vi "Build Channel Group Info.vi"(8 "Channel Data Reference":i32, 9 "Channel Groups in":T2(array[cluster]), 10 "Group Name":string, 11 "Channel Type":T1=enum."Input/Read") -> (0 "Group Index":i32, 1 "Channel Groups out":T2(array[cluster]))   [LabVIEW 2026, in "NIDMM Deployment Hooks.lvlib"]
uses:
  NIDMM Deployment Hooks.lvlib
  Types/Channel Mode.ctl
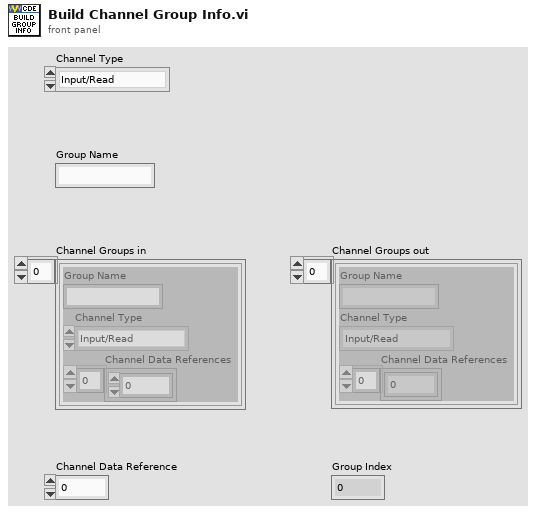
[diagram p1: front panel]
types:
  T1 = typedef "NIDMM Deployment Hooks.lvlib/Channel Mode.ctl" = enum16{"Output/Write", "Input/Read", "Input/ReadWrite"}
  T2 = cluster{"Group Name":string, "Channel Type":T1, "Channel Data References":i32[]}[]
  T3 = cluster{"Group Name":string, "Channel Type":T1, i32[]}
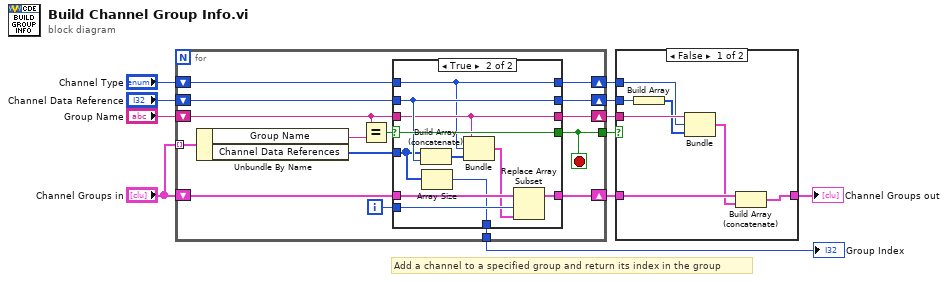
[diagram p0: block diagram]
diagram:
  # "Add a channel to a specified group and return its index in the group"
  n1 = for {
    tunnel: "Channel Groups in" -> [w26] mode=indexing
    shift-right: [w19] -> w8
    shift-left: "Channel Groups in" -> [w24]
    tunnel: [w17] -> w7
    shift-right: [w16] -> w11
    shift-left: "Channel Data Reference" -> [w22]
    shift-right: [w15] -> w10
    shift-left: "Group Name" -> [w20]
    shift-right: [w13] -> w2
    shift-left: "Channel Type" -> [w14]
    tunnel: [w12] -> w1
    i -> [w21]
    stop <- w17 stop-if-true
    n2 = Unbundle By Name(w26) -> ("Group Name"=w25:string, "Channel Data References"=w23:i32[])
    n3 = Equal?(x=w20, y=w25) -> (x = y?=w18:bool)
    n4 = case shown="True" w18 {
      selector: w18 -> [w30 w38]
      tunnel: w24 -> [w31 w42]
      tunnel: w23 -> [_ w33]
      tunnel: w22 -> [w29 w37]
      tunnel: w21 -> [_ w41]
      tunnel: w20 -> [w28 w36]
      tunnel: [w31 w39] -> w19
      tunnel: [w30 w38] -> w17
      tunnel: [w29 w37] -> w16
      tunnel: [w28 w36] -> w15
      tunnel: w14 -> [w27 w35]
      tunnel: [w27 w35] -> w13
      tunnel: [_ w32] -> w12
      frame False {
      }
      frame True {
        n5 = Build Array (concatenate)(w33, w37) -> (w34:i32[])
        n6 = Array Size(array=w33) -> (size(s)=w32:i32)
        n7 = Bundle("Group Name"=w36, "Channel Type"=w35, w34) -> (w40:T3)  [unwired: 1 in]
        n8 = Replace Array Subset(array=w42, new element=w40, index=w41) -> (w39:T2)
      }
    }
  }
  "Group Index" <- w1
  n9 = case shown="False" w7 {
    tunnel: w8 -> [w49 w50]
    tunnel: [w45 w50] -> w9
    tunnel: w10 -> [w48 _]
    tunnel: w11 -> [w47 _]
    tunnel: w2 -> [w44 _]
    frame False {
      n10 = Build Array(w47) -> (w43:i32[])
      n11 = Bundle("Group Name"=w48, "Channel Type"=w44, w43) -> (w46:T3)  [unwired: 1 in]
      n12 = Build Array (concatenate)(w49, w46) -> (w45:T2)
    }
    frame True {
    }
  }
  "Channel Groups out" <- w9
